vi "Configure Acquisition.vi"(0 "fpga interface in":refnum<k20>, 5 "continuous acquisition (T)":bool=TRUE, 7 "acquisition duration (s)":dbl, 11 "error in (no error)":errorcluster) -> (4 "fpga interface out":refnum<k20>, 15 "error out":errorcluster)   [LabVIEW 2023, in "GettingStarted_Acq_148X_Host.lvlib"]
uses:
  GettingStarted_Acq_148X_Host.lvlib
  Types/148x_Acq_FPGA_Reference.ctl
  <vilib>/Utility/error.llb/Error Cluster From Error Code.vi
  <vilib>/rvi/errors/niLvFpgaAdjustHostInterfaceError.vi
  <vilib>/rvi/interface/nirviReadWriteControl/nirviReadWriteControl.xnode
  NiFpgaLv.dll
  <vilib>/rvi/interface/Simulation/niFpgaSimulationCallBeginRW.vi
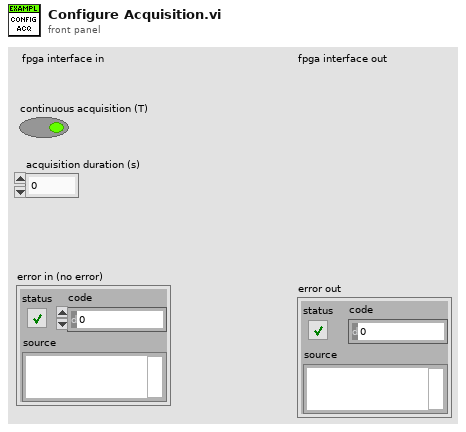
[diagram p1: front panel]
types:
  T1 = typedef "GettingStarted_Acq_148X_Host.lvlib/148x_Acq_FPGA_Reference.ctl" = refnum<k20>
  T2 = cluster{"continuous acquisition":bool, "acquisition duration (cycles)":u64}
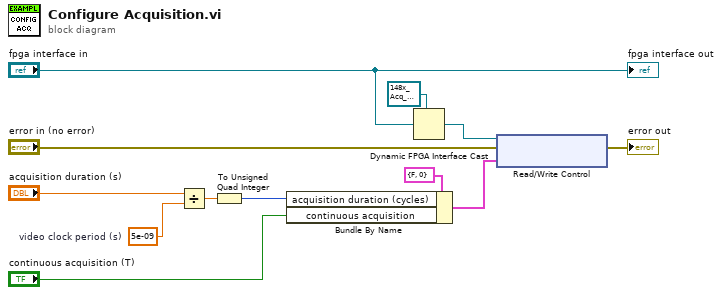
[diagram p0: block diagram]
diagram:
  w1 = 5e-09  # video clock period (s)
  n1 = Divide(x="acquisition duration (s)", y=w1) -> (x/y=w4:dbl)
  n2 = To Unsigned Quad Integer(1:w4) -> (0:w2:u64)
  n3 = Bundle By Name(cluster=T2 {"continuous acquisition"=FALSE, "acquisition duration (cycles)"=0} ("global acq config"), "acquisition duration (cycles)"=w2, "continuous acquisition"="continuous acquisition (T)") -> (w8:T2)
  n4 = Dynamic FPGA Interface Cast(Session In=T1 refnum ("FPGA VI Reference Out"), Type="fpga interface in") -> (Session Out=w6:T1)
  n5 = xnode "Read/Write Control"("FPGA VI Reference In"=w6, "error in"="error in (no error)", "global acq config"=w8) -> ("error out"=→"error out":errorcluster)  [unwired: 1 out]
  "fpga interface out" <- "fpga interface in"
